vi "Register Main View.vi"(11 "Message Enqueuer in":refnum<class "Message Enqueuer.lvclass">) -> (3 "Message Enqueuer out":refnum<class "Message Enqueuer.lvclass">)   [LabVIEW 2013]
uses:
  <vilib>/ActorFramework/Message Enqueuer/Message Enqueuer.lvclass
  <vilib>/ActorFrameworkMVC/View Observer/Registration Message/Registration Message.lvclass
  <vilib>/ActorFrameworkMVC/View Observer/Data Message/Data Message.lvclass
  Models/Main Model Messages/Register Project Number Msg/Register Project Number Msg.lvclass
  Views/Main View Messages/Project Number Msg/Project Number Msg.lvclass
  Models/Main Model Messages/Register Sensor Number Msg/Register Sensor Number Msg.lvclass
  Views/Main View Messages/Sensor Number Msg/Sensor Number Msg.lvclass
  <vilib>/ActorFrameworkMVC/UI Controller Messages/Subscribe View to Model Msg/Subscribe View to Model Msg.lvclass/Subscribe View to Model Msg.ctl
  <vilib>/ActorFramework/Message Enqueuer/Message Enqueuer.lvclass/Message Enqueuer.ctl
  <vilib>/ActorFramework/Message Enqueuer/Enqueue.vi
  <vilib>/ActorFramework/Message Priority Queue/Priority Enqueue.vi
  <vilib>/ActorFrameworkMVC/UI Controller Messages/Subscribe View to Model Msg/Subscribe View to Model Msg.lvclass
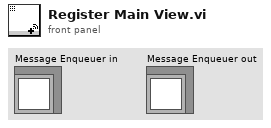
[diagram p1: front panel]
types:
  T1 = cluster{"Registration Message":string, "Data Message":string}[]
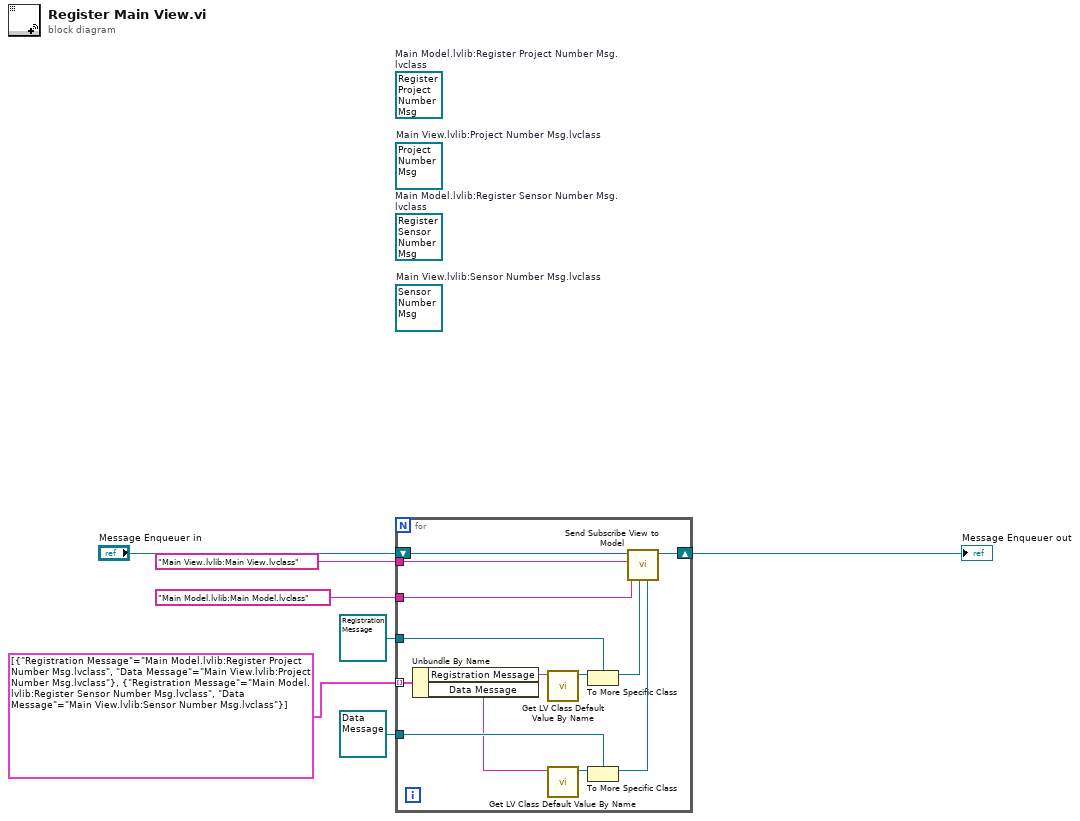
[diagram p0: block diagram]
diagram:
  (unwired) refnum<class "Sensor Number Msg.lvclass"> refnum  # Main View.lvlib:Sensor Number Msg.lvclass
  (unwired) refnum<class "Register Sensor Number Msg.lvclass"> refnum  # Main Model.lvlib:Register Sensor Number Msg.lvclass
  (unwired) refnum<class "Project Number Msg.lvclass"> refnum  # Main View.lvlib:Project Number Msg.lvclass
  (unwired) refnum<class "Register Project Number Msg.lvclass"> refnum  # Main Model.lvlib:Register Project Number Msg.lvclass
  n1 = for {
    tunnel: "Main View.lvlib:Main View.lvclass" ("View Name") -> [w19]
    tunnel: "Main Model.lvlib:Main Model.lvclass" ("Model Name") -> [w18]
    shift-right: [w17] -> w6
    shift-left: "Message Enqueuer in" -> [w20]
    tunnel: refnum<class "Registration Message.lvclass"> refnum ("Registration Message") -> [w14]
    tunnel: refnum<class "Data Message.lvclass"> refnum ("Data Message") -> [w13]
    tunnel: T1 [{"Registration Message"="Main Model.lvlib:Register Project Number Msg.lvclass", "Data Message"="Main View.lvlib:Project Number Msg.lvclass"}, {"Registration Message"="Main Model.lvlib:Register Sensor Number Msg.lvclass", "Data Message"="Main View.lvlib:Sensor Number Msg.lvclass"}] -> [w12] mode=indexing
    n2 = Unbundle By Name(w12) -> ("Registration Message"=w9:string, "Data Message"=w8:string)
    n3 = call <vilib>:"Get LV Class Default Value By Name.vi"("class name"=w9) -> ("object"=w16:refnum<class>)  [unwired: 9 in, 1 out]
    n4 = call <vilib>:"Get LV Class Default Value By Name.vi"("class name"=w8) -> ("object"=w15:refnum<class>)  [unwired: 9 in, 1 out]
    n5 = To More Specific Class(target class=w14, reference=w16) -> (specific class reference=w11:refnum<class "Registration Message.lvclass">)  [unwired: 1 in, 1 out]
    n6 = To More Specific Class(target class=w13, reference=w15) -> (specific class reference=w10:refnum<class "Data Message.lvclass">)  [unwired: 1 in, 1 out]
    n7 = call <vilib>:"Send Subscribe View to Model.vi"("Data Message"=w10, "Registration Message"=w11, "Model Name"=w18, "View Name"=w19, "Message Enqueuer"=w20) -> ("Message Enqueuer out"=w17:refnum<class "Message Enqueuer.lvclass">)  [unwired: 5 in, 1 out]
  }
  "Message Enqueuer out" <- w6
